vi "Write_Data.vi"(8 "error in (no error)":errorcluster caption="entrée d'erreur (pas d'erreur)", 10 "fields":T1={"Result"={"booleanValue"=FALSE}, "CreationDate"={"timestampValue"=""}, "Batch"={"stringValue"=""}, "SerialNumber"={"stringValue"=""}, "EndOfProduction"={"timestampValue"=""}, "FW_Version"={"mapValue"={"fields"={"Bootloader"={"mapValue"={"fields"={"File_Name"={"stringValue"=""}, "Version"={"mapValue"={"fields"={"Major"={"stringValue"=""}, "Minor"={"stringValue"=""}}}}, "Checksum"={"stringValue"=""}}}}, "SoftDevice"={"mapValue"={"fields"={"File_Name"={"stringValue"=""}, "Version"={"mapValue"={"fields"={"Major"={"stringValue"=""}, "Minor"={"stringValue"=""}}}}, "Checksum"={"stringValue"=""}}}}, "DFU"={"mapValue"={"fields"={"File_Name"={"stringValue"=""}, "Version"={"mapValue"={"fields"={"Major"={"stringValue"=""}, "Minor"={"stringValue"=""}}}}, "Checksum"={"stringValue"=""}}}}}}}, "PartNumber"={"stringValue"=""}, "OrderNumber"={"stringValue"="5"}, "Operator"={"stringValue"=""}, "AssembledProductName"={"stringValue"=""}}, 11 "Firebase PCBA en entrée":refnum<class "Firebase AssembledProducts.lvclass">) -> (0 "error out":errorcluster caption="sortie d'erreur", 3 "Firebase PCBA en sortie":refnum<class "Firebase AssembledProducts.lvclass">)   [LabVIEW 2020, in "Library Instrument & Equipement.lvlib" / "Library FireBase.lvlib" / "Firebase AssembledProducts.lvclass"]
doc: "Create New document\nPlease initialise the following values\n - Name BDD\n - Document\n - API Key"
uses:
  Firebase AssembledProducts.lvclass
  Firebase AssembledProducts.lvclass/Firebase AssembledProducts.ctl
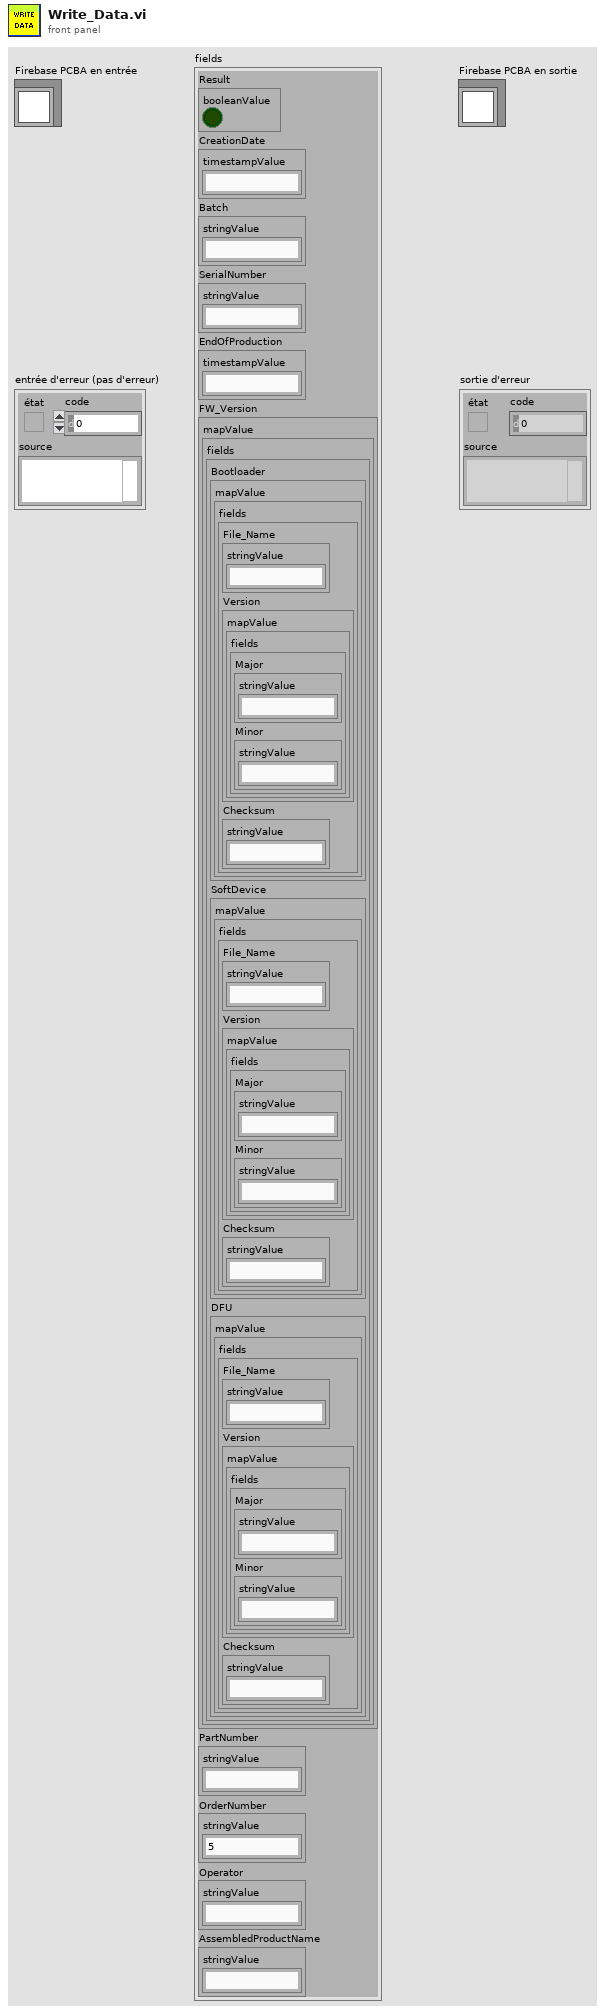
[diagram p1: front panel]
types:
  T1 = cluster{"Result":cluster{"booleanValue":bool}, "CreationDate":cluster{"timestampValue":string}, "Batch":cluster{"stringValue":string}, "SerialNumber":cluster{"stringValue":string}, "EndOfProduction":cluster{"timestampValue":string}, "FW_Version":cluster{"mapValue":cluster{"fields":cluster{"Bootloader":cluster{"mapValue":cluster{"fields":cluster{"File_Name":cluster{"stringValue":string}, "Version":cluster{"mapValue":cluster{"fields":cluster{"Major":cluster{"stringValue":string}, "Minor":cluster{"stringValue":string}}}}, "Checksum":cluster{"stringValue":string}}}}, "SoftDevice":cluster{"mapValue":cluster{"fields":cluster{"File_Name":cluster{"stringValue":string}, "Version":cluster{"mapValue":cluster{"fields":cluster{"Major":cluster{"stringValue":string}, "Minor":cluster{"stringValue":string}}}}, "Checksum":cluster{"stringValue":string}}}}, "DFU":cluster{"mapValue":cluster{"fields":cluster{"File_Name":cluster{"stringValue":string}, "Version":cluster{"mapValue":cluster{"fields":cluster{"Major":cluster{"stringValue":string}, "Minor":cluster{"stringValue":string}}}}, "Checksum":cluster{"stringValue":string}}}}}}}, "PartNumber":cluster{"stringValue":string}, "OrderNumber":cluster{"stringValue":string}, "Operator":cluster{"stringValue":string}, "AssembledProductName":cluster{"stringValue":string}}
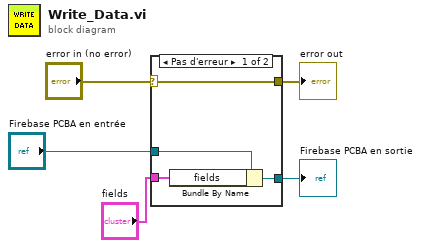
[diagram p0: block diagram]
diagram:
  n1 = case shown="Pas d'erreur" "error in (no error)" {
    selector: "error in (no error)" -> [w6 w11]
    tunnel: [w6 w11] -> w4
    tunnel: [w9 w10] -> w2
    tunnel: "Firebase PCBA en entrée" -> [w7 w10]
    tunnel: "fields" -> [w8 _]
    frame No Error {
      n2 = Bundle By Name(cluster=w7, "fields"=w8) -> (w9:refnum<class "Firebase AssembledProducts.lvclass">)
    }
    frame Error {
    }
  }
  "error out" <- w4
  "Firebase PCBA en sortie" <- w2
